vi "Set UI Update Timer.vi"(8 "error in (no error)":errorcluster, 11 "CIF_UI in":refnum<class "CIF_Manager_UI.lvclass">) -> (0 "error out":errorcluster, 3 "CIF_UI out":refnum<class "CIF_Manager_UI.lvclass">)   [LabVIEW 2021, in "CIF_Manager_UI.lvclass"]
uses:
  CIF_Manager_UI.lvclass
  C:/Program Files/National Instruments/LabVIEW 2021/vi.lib/CIF Foundation/CIF Core/CIFUI/CIF_UI.lvclass
  <vilib>/CIF Foundation/CIF Core/CIFUI/CIF_UI.lvclass/CIF_UI.ctl
  <vilib>/CIF Foundation/CIF Core/CIFUI/Accessors/Write Run Command Timer.vi
  CIF_Manager_UI.lvclass/CIF_Manager_UI.ctl
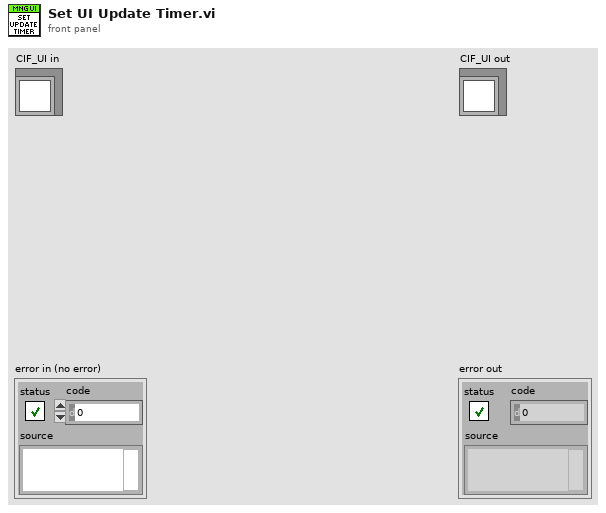
[diagram p1: front panel]
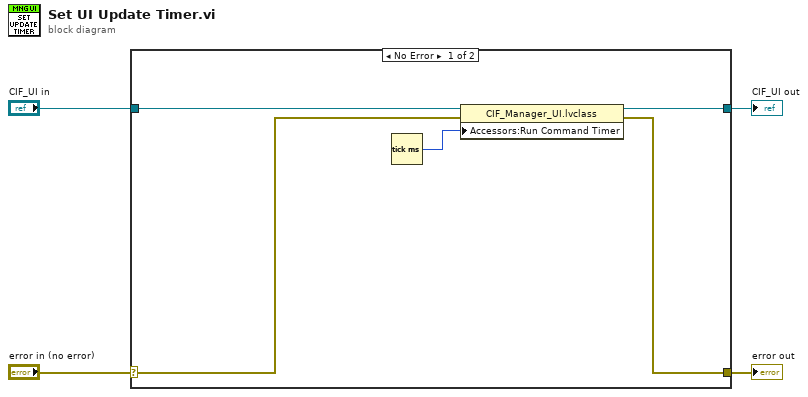
[diagram p0: block diagram]
diagram:
  n1 = case shown="No Error" "error in (no error)" {
    selector: "error in (no error)" -> [w6 w11]
    tunnel: [w5 w11] -> w3
    tunnel: [w8 w10] -> w1
    tunnel: "CIF_UI in" -> [w9 w10]
    frame No Error {
      n2 = Tick Count (ms)() -> (millisecond timer value=w7:u32)
      n3 = property class="CIF_Manager_UI.lvclass"(reference=w9, error in=w6, "Accessors:Run Command Timer"=w7) -> (reference out=w8:refnum<class "CIF_Manager_UI.lvclass">, error out=w5:errorcluster)
    }
    frame Error {
    }
  }
  "error out" <- w3
  "CIF_UI out" <- w1
